vi "cali_array upside down.vi"(10 "cali array in":dbl[][](array[numeric])) -> (2 "cali array out":dbl[][](array[numeric]))   [LabVIEW 2017]
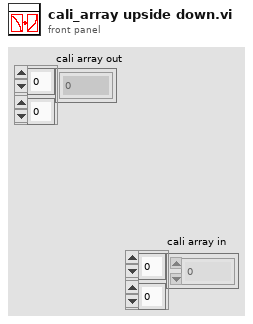
[diagram p1: front panel]
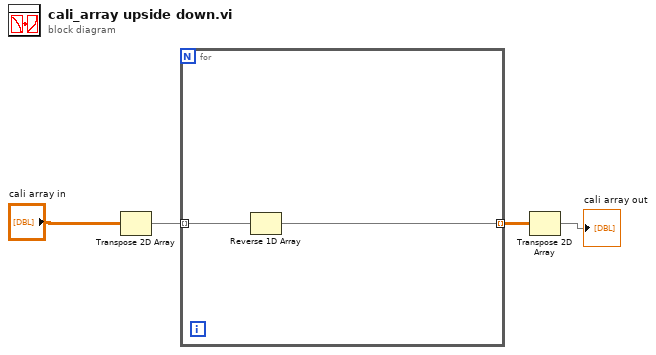
[diagram p0: block diagram]
diagram:
  n1 = Transpose 2D Array(2D array="cali array in") -> (transposed array=w4:dbl[][])
  n2 = for {
    tunnel: w4 -> [w6] mode=indexing
    tunnel: [w5] -> w3 mode=indexing
    n3 = Reverse 1D Array(array=w6) -> (reversed array=w5:dbl[])
  }
  n4 = Transpose 2D Array(2D array=w3) -> (transposed array=→"cali array out":dbl[][])
